vi "niRFUtil TRC Save Traces to File.vi"   [LabVIEW 2015, in "niRFUtil.lvlib"]
uses:
  niRFUtil.lvlib
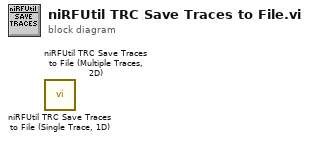
[diagram p0: block diagram]
diagram:
  n1 = call "niRFUtil TRC Save Traces to File (Single Trace, 1D).vi"() -> ()  [unwired: 15 in, 1 out]
  n2 = call "niRFUtil TRC Save Traces to File (Multiple Traces, 2D).vi"() -> ()  [unwired: 15 in, 1 out]
